vi "visa_status.vi"(8 "error in (no error)":errorcluster) -> ()   [LabVIEW 2016]
uses:
  <vilib>/Utility/error.llb/DialogType.ctl
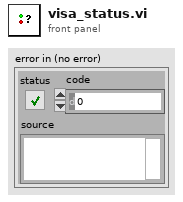
[diagram p1: front panel]
types:
  T1 = typedef "DialogType.ctl" = u16
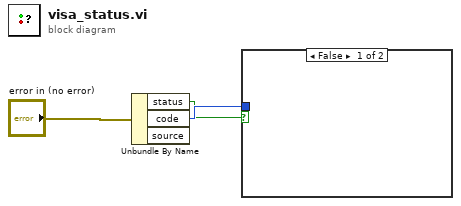
[diagram p0: block diagram]
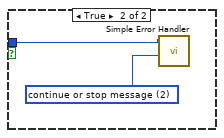
[diagram p2: hidden frame]
diagram:
  n1 = Unbundle By Name("error in (no error)") -> ("status"=w2:bool, "code"=w3:i32)  [unwired: 1 out]
  n2 = case shown="False" w2 {
    tunnel: w3 -> [_ w5]
    frame False {
    }
    frame True {
      w4 = T1 2 items=["no dialog", "OK message", "continue or stop message", "OK message + warnings", "continue/stop + warnings"] ("type of dialog (OK msg:1)")
      n3 = call <vilib>:"Simple Error Handler.vi"("error code (no error:0)"=w5, "type of dialog (OK msg:1)"=w4) -> ()  [unwired: 3 in, 5 out]
    }
  }
